vi "Build RT Data Cluster.vi"(0 "Device Reference in":T1 format="%.0x", 2 "RT Data in":T2={"Device ref"=0, "Scan Period (uSec)"=10000, "Device Channels"={"Status"={"BD Refs"=[], "Length"=0, "FIFO Index"=0, "Data"=[]}, "Command"={"BD Refs"=[], "Data"=[], "Length"=0, "FIFO Index"=0}}, "Local Chassis"=[], "EtherCAT Masters"=[], "Async"={"Status"=refnum, "Command"=refnum, "Input FIFO"=refnum, "Input FIFO buffer"=[], "Output FIFO"=refnum, "Output FIFO buffer"=[], "Async VI Ref"=refnum}, "ECAT Reconfig"={"Reconfig Module Found"=FALSE, "VI Ref"=refnum, "Status"=refnum}, "Device Error"={"status"=FALSE, "code"=0, "source"=""}, "DeviceName"="", "PCLSync?"=FALSE} {"Device Channels"."Status"."BD Refs"."Data Reference" format="%.0x"; "Device Channels"."Command"."BD Refs"."Data Reference" format="%.0x"; "Local Chassis"."FPGA"."VS ref" format="%.0x"; "Local Chassis"."RSI Modules"."VS ref" format="%.0x"; "Local Chassis"."VS ref" format="%.0x"; "Device ref" format="%.0x"; "EtherCAT Masters"."Generic EtherCAT Slaves"."VS ref" format="%.0x"; "EtherCAT Masters"."VS ref" format="%.0x"; "EtherCAT Masters"."EtherCAT Slaves"."FPGA"."VS ref" format="%.0x"; "EtherCAT Masters"."EtherCAT Slaves"."RSI Modules"."VS ref" format="%.0x"; "EtherCAT Masters"."EtherCAT Slaves"."VS ref" format="%.0x"}, 3 "error in":errorcluster) -> (7 "RT Data out":T2={"Device ref"=0, "Scan Period (uSec)"=10000, "Device Channels"={"Status"={"BD Refs"=[], "Length"=0, "FIFO Index"=0, "Data"=[]}, "Command"={"BD Refs"=[], "Data"=[], "Length"=0, "FIFO Index"=0}}, "Local Chassis"=[], "EtherCAT Masters"=[], "Async"={"Status"=refnum, "Command"=refnum, "Input FIFO"=refnum, "Input FIFO buffer"=[], "Output FIFO"=refnum, "Output FIFO buffer"=[], "Async VI Ref"=refnum}, "ECAT Reconfig"={"Reconfig Module Found"=FALSE, "VI Ref"=refnum, "Status"=refnum}, "Device Error"={"status"=FALSE, "code"=0, "source"=""}, "DeviceName"="", "PCLSync?"=FALSE} {"Device Channels"."Status"."BD Refs"."Data Reference" format="%.0x"; "Device Channels"."Command"."BD Refs"."Data Reference" format="%.0x"; "Local Chassis"."FPGA"."VS ref" format="%.0x"; "Local Chassis"."RSI Modules"."VS ref" format="%.0x"; "Local Chassis"."VS ref" format="%.0x"; "Device ref" format="%.0x"; "EtherCAT Masters"."Generic EtherCAT Slaves"."VS ref" format="%.0x"; "EtherCAT Masters"."VS ref" format="%.0x"; "EtherCAT Masters"."EtherCAT Slaves"."FPGA"."VS ref" format="%.0x"; "EtherCAT Masters"."EtherCAT Slaves"."RSI Modules"."VS ref" format="%.0x"; "EtherCAT Masters"."EtherCAT Slaves"."VS ref" format="%.0x"})   [LabVIEW 2015, in "Scan Engine Custom Device.lvlib"]
uses:
  Scan Engine Custom Device.lvlib
  Type Defs/RT Data.ctl
  <vilib>/NI Veristand/Custom Device API/Custom Device Item Ref.ctl
  Type Defs/Device Channels.ctl
  Type Defs/Output Data.ctl
  <vilib>/NI Veristand/Custom Device API/Block Data Reference.ctl
  <vilib>/NI Veristand/Custom Device API/Data Reference.ctl
  Type Defs/Input Data.ctl
  Type Defs/Local Chassis Data.ctl
  Type Defs/RSI Module Data.ctl
  Type Defs/Open Module IOVs.ctl
  Modules.lvlibp/RSI Module/RSI Module.lvclass
  Modules.lvlibp/RSI Module/Module Models.ctl
  Modules.lvlibp/RSI Module/Channel Type.ctl
  Type Defs/Module Config Data.ctl
  Type Defs/Mixed IO.ctl
  Type Defs/FPGA Data.ctl
  Type Defs/UDV Data.ctl
  Type Defs/UDV Data Type.ctl
  Type Defs/FXP Config.ctl
  Type Defs/Mod Size Indexes.ctl
  Type Defs/EtherCAT Master Data.ctl
  Type Defs/EtherCAT Slave Data.ctl
  Type Defs/Generic ECAT Slave RT-Data-Array.ctl
  Type Defs/Generic ECAT Slave Data Cluster.ctl
  Type Defs/Generic ECAT Slave IOV Cluster.ctl
  Type Defs/Async Data.ctl
  Type Defs/Async Status.ctl
  Type Defs/Async State.ctl
  Type Defs/Async Command.ctl
  Type Defs/ECAT Reconfig Data.ctl
  Type Defs/ECAT Reconfig Status.ctl
  Type Defs/ECAT Reconfig State.ctl
  Type Defs/Data Ref FGV Command.ctl
  <vilib>/NIScanEngine/ConfigurableFaults/Fault Desc Control.ctl
  Globals/Property Strings.vi
  Globals/RT Globals.vi
  Globals/String Constants.vi
  <vilib>/NI Veristand/Custom Device API/Get Item Property (U16).vi
  <vilib>/NI Veristand/Custom Device API/Get Item Property (U32).vi
  <vilib>/NI Veristand/Custom Device API/Custom Device API.lvlib
  <vilib>/NI Veristand/Custom Device Tools/Custom Device Utility Library/Custom Device Utility Library.lvlib
  <vilib>/NIScanEngine/ConfigurableFaults/Config Faults.lvlib
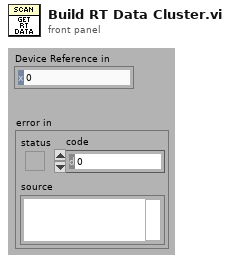
[diagram p1: front panel]
types:
  T1 = typedef "Custom Device API.lvlib/Custom Device Item Ref.ctl" = u64
  T2 = typedef "Scan Engine Custom Device.lvlib/RT Data.ctl" = cluster{"Device ref":T1, "Scan Period (uSec)":u32, "Device Channels":T3, "Local Chassis":T8[], "EtherCAT Masters":T20[], "Async":T25, "ECAT Reconfig":T26, "Device Error":errorcluster, "DeviceName":string, "PCLSync?":bool}
  T3 = typedef "Scan Engine Custom Device.lvlib/Device Channels.ctl" = cluster{"Status":T4, "Command":T7}
  T4 = typedef "Scan Engine Custom Device.lvlib/Output Data.ctl" = cluster{"BD Refs":T5[], "Length":i32, "FIFO Index":i32, "Data":dbl[]}
  T5 = typedef "Custom Device API.lvlib/Block Data Reference.ctl" = cluster{"Data Reference":T6, "Offset":u64, "Length":u64}
  T6 = typedef "Custom Device API.lvlib/Data Reference.ctl" = i32
  T7 = typedef "Scan Engine Custom Device.lvlib/Input Data.ctl" = cluster{"BD Refs":T5[], "Data":dbl[], "Length":i32, "FIFO Index":i32}
  T8 = typedef "Scan Engine Custom Device.lvlib/Local Chassis Data.ctl" = cluster{"VS ref":T1, "RSI Modules":T9[], "FPGA":T15[], "Input Mod Size Idxs":T19, "Output Modules":i32[], "MixedIO Mod Size Idxs":T19}
  T9 = typedef "Scan Engine Custom Device.lvlib/RSI Module Data.ctl" = cluster{"VS ref":T1, "IOV ref":refnum<k21>, "Open Mod refs":T10, "Module DVR":refnum<data-value>, "Slot":u32, "Model":T11, "Channel Type":T12, "EtherCAT?":bool, "CDInput Data":T7, "CDOutput Data":T4, "Module Config Data":T13, "Mixed IO":T14}
  T10 = typedef "Scan Engine Custom Device.lvlib/Open Module IOVs.ctl" = cluster{"Analog Read":refnum<k21>, "Digital Read":refnum<k21>, "Analog Write":refnum<k21>, "Digital Write":refnum<k21>}
  T11 = typedef "Modules.lvlibp/RSI Module.lvclass/Module Models.ctl" = enum16{"Empty", "NI 9201", "NI 9203", "NI 9205", "NI 9206", "NI 9207", "NI 9208", "NI 9211", "NI 9212", "NI 9213", "NI 9214", "NI 9215", "NI 9217", "NI 9219", "NI 9220", "NI 9221", "NI 9222", "NI 9223", "NI 9225", "NI 9227", "NI 9229", "NI 9233", "NI 9234", "NI 9235", "NI 9236", "NI 9237", "NI 9239", "NI 9242", "NI 9244", "NI 9263", "NI 9264", "NI 9265", "NI 9269", "NI 9375", "NI 9401", "NI 9402", "NI 9403", "NI 9411", "NI 9421", "NI 9422", "NI 9423", "NI 9425", "NI 9426", "NI 9435", "NI 9437", "NI 9472", "NI 9474", "NI 9475", "NI 9476", "NI 9477", "NI 9478", "NI 9481", "NI 9482", "NI 9485"}
  T12 = typedef "Modules.lvlibp/RSI Module.lvclass/Channel Type.ctl" = enum16{"Analog", "Digital"}
  T13 = typedef "Scan Engine Custom Device.lvlib/Module Config Data.ctl" = cluster{"Configurable?":bool, "Config Block Data Refs":T5[], "Config Data DVR":refnum<data-value>, "Previous Values":dbl[], "Local Reconfig VI Ref":refnum<vi>}
  T14 = typedef "Scan Engine Custom Device.lvlib/Mixed IO.ctl" = cluster{"Input Channel Indices":i32[], "Input Buffer":dbl[]}
  T15 = typedef "Scan Engine Custom Device.lvlib/FPGA Data.ctl" = cluster{"VS ref":T1, "IOV ref":refnum<k21>, "FPGA Target":enum16{"Local", "EtherCAT"}, "Product Code":u32, "Bitfile Signature":string, "Bitfile Path (RT)":path, "FPGA Session":u32, "Input Data":T7, "Output Data":T4, "UDVs":cluster{"From FPGA":T16[], "To FPGA":T16[]}}
  T16 = typedef "Scan Engine Custom Device.lvlib/UDV Data.ctl" = cluster{"VS ref":T1, "IOV Ref":refnum<k21>, "Name":string, "UDV Data Type":T17, "Supported Type?":bool, "FXP Config":T18, "FXP VI Ref":refnum<vi>}
  T17 = typedef "Scan Engine Custom Device.lvlib/UDV Data Type.ctl" = enum16{"Boolean", "Fixed Point", "Int8", "Int16", "Int32", "Int64", "U32 Bit Field", "UInt8", "UInt16", "UInt32", "UInt64", "Other"}
  T18 = typedef "Scan Engine Custom Device.lvlib/FXP Config.ctl" = cluster{"signed":bool, "size":u32, "integersize":i32}
  T19 = typedef "Scan Engine Custom Device.lvlib/Mod Size Indexes.ctl" = cluster{"4":i32[], "8":i32[], "16":i32[], "32":i32[], "other":i32[]}
  T20 = typedef "Scan Engine Custom Device.lvlib/EtherCAT Master Data.ctl" = cluster{"VS ref":T1, "IOV ref":refnum<k21>, "Master ID":u32, "Cyclic Data Bandwidth":u32, "EtherCAT Slaves":T21[], "Generic EtherCAT Slaves":T22}
  T21 = typedef "Scan Engine Custom Device.lvlib/EtherCAT Slave Data.ctl" = cluster{"VS ref":T1, "IOV ref":refnum<k21>, "Position Address":u16, "RSI Modules":T9[], "FPGA":T15[], "Input Mod Size Idxs":T19, "Output Modules":i32[], "MixedIO Mod Size Idxs":T19}
  T22 = typedef "Scan Engine Custom Device.lvlib/Generic ECAT Slave RT-Data-Array.ctl" = T23[]
  T23 = typedef "Scan Engine Custom Device.lvlib/Generic ECAT Slave Data Cluster.ctl" = cluster{"VS ref":T1, "IOV ref":refnum<k21>, "Position Address":u16, "I/O Imput Vars ":T24[], "I/O Output Vars":T24[], "I/O Input Data":T7, "I/O Output Data":T4}
  T24 = typedef "Scan Engine Custom Device.lvlib/Generic ECAT Slave IOV Cluster.ctl" = cluster{"VS ref":T1, "IOV Ref":refnum<k21>, "Name":string, "UDV Data Type":T17}
  T25 = typedef "Scan Engine Custom Device.lvlib/Async Data.ctl" = cluster{"Status":refnum<queue>, "Command":refnum<queue>, "Input FIFO":refnum<k33>, "Input FIFO buffer":dbl[], "Output FIFO":refnum<k33>, "Output FIFO buffer":dbl[], "Async VI Ref":refnum<vi>}
  T26 = typedef "Scan Engine Custom Device.lvlib/ECAT Reconfig Data.ctl" = cluster{"Reconfig Module Found":bool, "VI Ref":refnum<vi>, "Status":refnum<queue>}
  T27 = typedef "Config Faults.lvlib/Fault Desc Control.ctl" = cluster{"code":i32, "level or level before threshold":i32, "occurrence threshold":u32, "time window in seconds":u32, "level after threshold":i32}
  T28 = typedef "Scan Engine Custom Device.lvlib/Data Ref FGV Command.ctl" = enum16{"Intialize", "Get", "Update"}
  T29 = typedef "Fault.ctl" = cluster{"code":i32, "level":i32, "first reported time":timestamp, "number reported":u32}
  T30 = typedef "Custom Device API.lvlib/Custom Device Channel.ctl" = cluster{"Type":T31, "Units":string, "Default Value":dbl, "Faultable":bool, "Scalable":bool}
  T31 = typedef "Custom Device API.lvlib/Custom Device Channel Type.ctl" = enum16{"Input", "Output"}
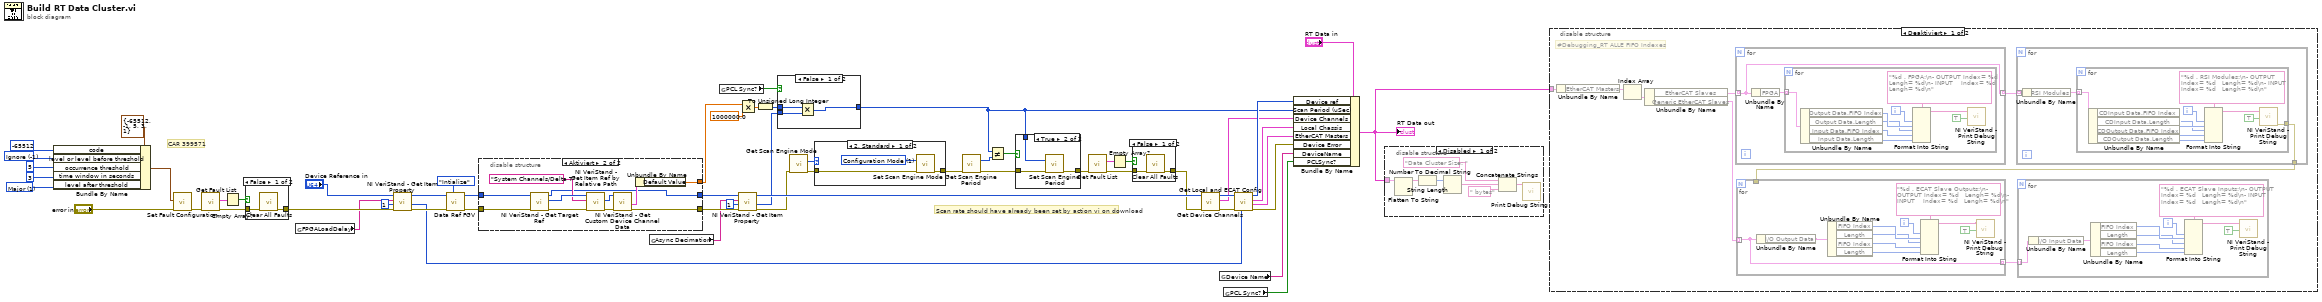
[diagram p0: block diagram]
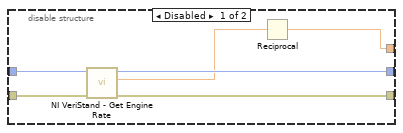
[diagram p9: hidden frame]
diagram:
  w14 = -1 items=["Ignore"=-1, "Minor"=0, "Major"=1] ("level or level before threshold")
  w17 = 1 items=["Ignore"=-1, "Minor"=0, "Major"=1] ("level after threshold")
  # "CAR 399571"
  # "Scan rate should have already been set by action vi on download"
  n1 = Bundle By Name(cluster=T27 {"code"=-65512, "level or level before threshold"=-1, "occurrence threshold"=5, "time window in seconds"=3, "level after threshold"=1} ("fault configuration"), "code"=-65512, "level or level before threshold"=w14, "occurrence threshold"=u32 5, "time window in seconds"=u32 3, "level after threshold"=w17) -> (w18:T27)
  n2 = call <vilib>:"Set Fault Configuration.vi"("error in (no error)"="error in", "fault configuration"=w18) -> ("error out"=w12:errorcluster)  [unwired: 7 in]
  n3 = call <vilib>:"Get Fault List.vi"("error in (no error)"=w12) -> ("error out"=w23:errorcluster, "fault list"=w21:T29[])  [unwired: 9 in]
  n4 = Empty Array?(array=w21) -> (empty?=w22:bool)
  n5 = case shown="False" w22 {
    tunnel: w23 -> [w59 w60]
    tunnel: [w58 w60] -> w20
    frame False {
      n6 = call <vilib>:"Clear All Faults.vi"("error in (no error)"=w59) -> ("error out"=w58:errorcluster)  [unwired: 10 in]
    }
    frame True {
    }
  }
  n7 = global read "Property Strings.vi" "FPGALoadDelay"() -> (w5:string)
  n8 = call-poly <vilib>:"NI VeriStand - Get Item Property.vi"("error in (no error)"=w20, "Default Value"=u16 1, "Property Name"=w5, "Item Ref in"="Device Reference in") -> ("error out"=w8:errorcluster, "Value"=w2:u16, "Item Ref out"=w6:T1)  [unwired: 4 in, 1 out]
  n9 = call "Data Ref FGV.vi"("Command"=Data_Ref_FGV_Command."Intialize", "error in (no error)"=w8, "Device Ref in"=w6) -> ("error out"=w57:errorcluster, "Device Ref out"=w56:T1)  [unwired: 5 in, 2 out]
  n10 = disable-structure shown="Aktiviert" {
    disable-tunnel: [w61 w68] -> w51
    disable-tunnel: [w66 w67] -> w45
    disable-tunnel: [w65 w69] -> w46
    disable-tunnel: w57 -> [w64 w76]
    disable-tunnel: w56 -> [w63 w77]
    frame Disabled {
      n11 = call <vilib>:"NI VeriStand - Get Engine Rate.vi"("error in (no error)"=w64, "Item Ref in"=w63) -> ("error out"=w66:errorcluster, "Rate (Hz)"=w62:dbl, "Item Ref out"=w65:T1)  [unwired: 7 in]
      n12 = Reciprocal(x=w62) -> (1/x=w61:dbl)
    }
    frame Enabled {
      n13 = call <vilib>:"NI VeriStand - Get Target Ref.vi"("error in"=w76, "Item Ref in"=w77) -> ("error out"=w74:errorcluster, "Target Ref"=w75:T1, "Item Ref out"=w69:T1)  [unwired: 6 in, 1 out]
      n14 = call <vilib>:"NI VeriStand - Get Item Ref by Relative Path.vi"("error in"=w74, "Relative Item Path"="System Channels/Delta T", "Section Ref in"=w75) -> ("error out"=w71:errorcluster, "Item Ref"=w72:T1)  [unwired: 5 in, 2 out]
      n15 = call <vilib>:"NI VeriStand - Get Custom Device Channel Data.vi"("error in (no error)"=w71, "Channel Ref in"=w72) -> ("error out"=w67:errorcluster, "Channel"=w70:T30)  [unwired: 4 in, 4 out]
      n16 = Unbundle By Name(w70) -> ("Default Value"=w68:dbl)
    }
  }
  n17 = global read "Property Strings.vi" "Async Decimation"() -> (w43:string)
  n18 = global read "RT Globals.vi" "PCL Sync?"() -> (w40:bool)
  n19 = call-poly <vilib>:"NI VeriStand - Get Item Property.vi"("error in (no error)"=w45, "Default Value"=u32 1, "Property Name"=w43, "Item Ref in"=w46) -> ("error out"=w31:errorcluster, "Value"=w41:u32, "Item Ref out"=w44:T1)  [unwired: 4 in, 1 out]
  n20 = Multiply(x=w51, y=1000000.0) -> (x*y=w25:dbl)
  n21 = To Unsigned Long Integer(number=w25) -> (unsigned 32bit integer=w24:u32)
  n22 = case shown="False" w40 {
    tunnel: w24 -> [w80 w81]
    tunnel: w41 -> [w79 _]
    tunnel: [w78 w81] -> w26
    frame False {
      n23 = Multiply(x=w80, y=w79) -> (x*y=w78:u32)
    }
    frame True {
    }
  }
  n24 = call <vilib>:"Get Scan Engine Mode.vi"("error in (no error)"=w31) -> ("error out"=w33:errorcluster, "mode"=w32:i32)  [unwired: 9 in]
  n25 = case shown="2, Standard" w32 {
    tunnel: w33 -> [w83 w85]
    tunnel: [w82 w85] -> w30
    frame 2, Default {
      w84 = 1 items=["Configuration Mode"=1, "Active Mode"=2] ("mode (Active Mode)")
      n26 = call <vilib>:"Set Scan Engine Mode.vi"("mode (Active Mode)"=w84, "error in (no error)"=w83) -> ("error out"=w82:errorcluster)  [unwired: 13 in]
    }
    frame 1 {
    }
  }
  n27 = call <vilib>:"Get Scan Engine Period.vi"("error in (no error)"=w30) -> ("scan period (uSec)"=w29:u32, "error out"=w27:errorcluster)  [unwired: 13 in]
  n28 = Not Equal?(x=w26, y=w29) -> (x != y?=w28:bool)
  n29 = case shown="True" w28 {
    tunnel: [w86 w89] -> w35
    tunnel: w27 -> [w86 w88]
    tunnel: w26 -> [_ w87]
    frame False {
    }
    frame True {
      n30 = call <vilib>:"Set Scan Engine Period.vi"("scan period (uSec)"=w87, "error in (no error)"=w88) -> ("error out"=w89:errorcluster)  [unwired: 13 in]
    }
  }
  n31 = call <vilib>:"Get Fault List.vi"("error in (no error)"=w35) -> ("error out"=w38:errorcluster, "fault list"=w36:T29[])  [unwired: 9 in]
  n32 = Empty Array?(array=w36) -> (empty?=w37:bool)
  n33 = case shown="False" w37 {
    tunnel: w38 -> [w91 w92]
    tunnel: [w90 w92] -> w34
    frame False {
      n34 = call <vilib>:"Clear All Faults.vi"("error in (no error)"=w91) -> ("error out"=w90:errorcluster)  [unwired: 10 in]
    }
    frame True {
    }
  }
  n35 = call "Get Device Channels.vi"("error in"=w34, "Device Reference in"=w44) -> ("error out"=w49:errorcluster, "Device Channels"=w47:T3, "Device Reference out"=w48:T1)  [unwired: 7 in]
  n36 = global read "String Constants.vi" "Device Name"() -> (w10:string)
  n37 = global read "RT Globals.vi" "PCL Sync?"() -> (w9:bool)
  n38 = call "Get Local and ECAT Config.vi"("fpga wait (s)"=w2, "error in (no error)"=w49, "Device Reference in"=w48) -> ("error out"=w3:errorcluster, "ECAT Masters"=w39:T20[], "Local Chassis"=w55:T8[], "Device Reference out"=w53:T1)  [unwired: 5 in]
  n39 = Bundle By Name(cluster="RT Data in", "Device ref"=w53, "Scan Period (uSec)"=w26, "Device Channels"=w47, "Local Chassis"=w55, "EtherCAT Masters"=w39, "Device Error"=w3, "DeviceName"=w10, "PCLSync?"=w9) -> (w1:T2)
  "RT Data out" <- w1
  n40 = disable-structure shown="Disabled" {
    disable-tunnel: w1 -> [w93 _]
    frame Disabled {
      n41 = Flatten To String(anything=w93) -> (data string=w94:string)  [unwired: 3 in, 2 out]
      n42 = String Length(string=w94) -> (length=w96:i32)
      n43 = Number To Decimal String(number=w96) -> (decimal integer string=w97:string)  [unwired: 1 in]
      n44 = Concatenate Strings("Data Cluster Size: " ("string"), w97, " bytes" ("string")) -> (w99:string)
      n45 = call "Print Debug String.vi"("String to write"=w99) -> ()  [unwired: 9 in, 1 out]
    }
    frame Enabled {
    }
  }
  n46 = disable-structure shown="Deaktiviert" {
    disable-tunnel: w1 -> [w107 _]
    frame Disabled {
      # "#Debugging_RT ALLE FIFO Indexes"
      n47 = Unbundle By Name(w107) -> ("EtherCAT Masters"=w106:T20[])
      n48 = Index Array(array=w106) -> (element=w105:T20)  [unwired: 1 in]
      n49 = Unbundle By Name(w105) -> ("EtherCAT Slaves"=w104:T21[], "Generic EtherCAT Slaves"=w102:T22)
      n50 = for {
        tunnel: w104 -> [w141] mode=indexing
        tunnel: [w141] -> w103 mode=indexing
        n51 = Unbundle By Name(w141) -> ("FPGA"=w142:T15[])
        n52 = for {
          tunnel: w142 -> [w151] mode=indexing
          i -> [w147]
          n53 = Unbundle By Name(w151) -> ("Output Data.FIFO Index"=w146:i32, "Output Data.Length"=w145:i32, "Input Data.FIFO Index"=w144:i32, "Input Data.Length"=w143:i32)
          n54 = Format Into String(format string="%d . FPGA:\n- OUTPUT Index= %d   Lengh= %d\n- INPUT    Index= %d   Lengh= %d\n", w147, w146, w145, w144, w143) -> (resulting string=w150:string)  [unwired: 2 in, 1 out]
          n55 = call <vilib>:"NI VeriStand - Print Debug String.vi"("Add to log file? (T)"=TRUE, "Message"=w150) -> ()  [unwired: 9 in, 1 out]
        }
      }
      n56 = for {
        tunnel: w103 -> [w129] mode=indexing
        tunnel: [w128] -> w100
        n57 = Unbundle By Name(w129) -> ("RSI Modules"=w130:T9[])
        n58 = for {
          tunnel: w130 -> [w140] mode=indexing
          tunnel: [w131] -> w128
          i -> [w136]
          n59 = Unbundle By Name(w140) -> ("CDInput Data.FIFO Index"=w135:i32, "CDInput Data.Length"=w134:i32, "CDOutput Data.FIFO Index"=w133:i32, "CDOutput Data.Length"=w132:i32)
          n60 = Format Into String(format string="%d . RSI Modules:\n- OUTPUT Index= %d   Lengh= %d\n- INPUT    Index= %d   Lengh= %d\n", w136, w135, w134, w133, w132) -> (resulting string=w139:string)  [unwired: 2 in, 1 out]
          n61 = call <vilib>:"NI VeriStand - Print Debug String.vi"("Add to log file? (T)"=TRUE, "Message"=w139) -> ("error out"=w131:errorcluster)  [unwired: 9 in]
        }
      }
      n62 = for {
        tunnel: w102 -> [w118] mode=indexing
        tunnel: [w118] -> w101 mode=indexing
        tunnel: w100 -> [_]
        i -> [w124]
        n63 = Unbundle By Name(w118) -> ("I/O Output Data"=w119:T4)
        n64 = Unbundle By Name(w119) -> ("FIFO Index"=w123:i32, "Length"=w122:i32, "FIFO Index"=w121:i32, "Length"=w120:i32)
        n65 = Format Into String(format string="%d . ECAT Slave Outputs:\n- OUTPUT Index= %d   Lengh= %d\n- INPUT    Index= %d   Lengh= %d\n", w124, w123, w122, w121, w120) -> (resulting string=w127:string)  [unwired: 2 in, 1 out]
        n66 = call <vilib>:"NI VeriStand - Print Debug String.vi"("Add to log file? (T)"=TRUE, "Message"=w127) -> ()  [unwired: 9 in, 1 out]
      }
      n67 = for {
        tunnel: w101 -> [w108] mode=indexing
        i -> [w114]
        n68 = Unbundle By Name(w108) -> ("I/O Input Data"=w109:T7)
        n69 = Unbundle By Name(w109) -> ("FIFO Index"=w113:i32, "Length"=w112:i32, "FIFO Index"=w111:i32, "Length"=w110:i32)
        n70 = Format Into String(format string="%d . ECAT Slave Inputs:\n- OUTPUT Index= %d   Lengh= %d\n- INPUT    Index= %d   Lengh= %d\n", w114, w113, w112, w111, w110) -> (resulting string=w117:string)  [unwired: 2 in, 1 out]
        n71 = call <vilib>:"NI VeriStand - Print Debug String.vi"("Add to log file? (T)"=TRUE, "Message"=w117) -> ()  [unwired: 9 in, 1 out]
      }
    }
    frame Enabled {
    }
  }
